vi "Controls and Indicators.vi"(4 "Motors Enable":bool[](array[boolean])=[FALSE, FALSE, FALSE], 5 "Virtual Spring":dbl=0.3, 6 "Tension Control":bool=TRUE, 7 "Velocity Damping":dbl=0.01, 8 "Start, End Point":bool[](array[boolean]), 9 "Target Stop":bool, 10 "Encoder Initialize":bool, 11 "Trajectory":i32(slide) scale=0.0..2.0) -> ()   [LabVIEW 2021]
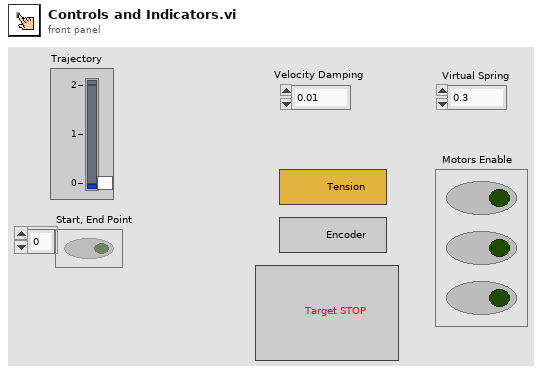
[diagram p1: front panel]
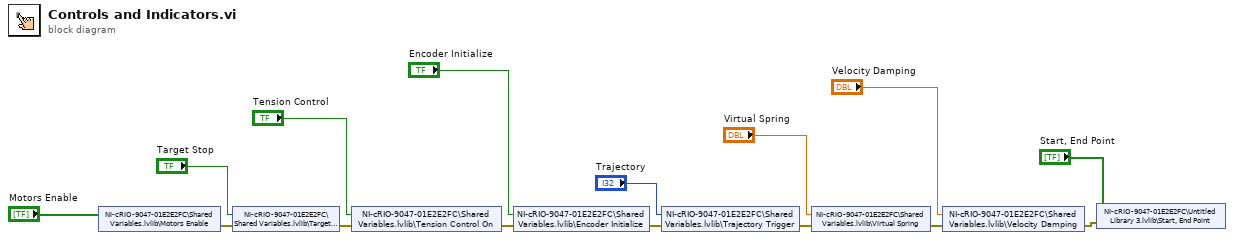
[diagram p0: block diagram]
diagram:
  n1 = shared-variable "NI-cRIO-9047-01E2E2FC\\Shared Variables.lvlib\\Motors Enable"("Motors Enable") -> (error out=w4:errorcluster)  [unwired: 1 in]
  n2 = shared-variable "NI-cRIO-9047-01E2E2FC\\Shared Variables.lvlib\\Target Stop"("Target Stop", error in=w4) -> (error out=w3:errorcluster)
  n3 = shared-variable "NI-cRIO-9047-01E2E2FC\\Shared Variables.lvlib\\Tension Control On"("Tension Control", error in=w3) -> (error out=w13:errorcluster)
  n4 = shared-variable "NI-cRIO-9047-01E2E2FC\\Shared Variables.lvlib\\Encoder Initialize"("Encoder Initialize", error in=w13) -> (error out=w14:errorcluster)
  n5 = shared-variable "NI-cRIO-9047-01E2E2FC\\Shared Variables.lvlib\\Trajectory Trigger"("Trajectory", error in=w14) -> (error out=w15:errorcluster)
  n6 = shared-variable "NI-cRIO-9047-01E2E2FC\\Shared Variables.lvlib\\Virtual Spring"("Virtual Spring", error in=w15) -> (error out=w12:errorcluster)
  n7 = shared-variable "NI-cRIO-9047-01E2E2FC\\Shared Variables.lvlib\\Velocity Damping"("Velocity Damping", error in=w12) -> (error out=w2:errorcluster)
  n8 = shared-variable "NI-cRIO-9047-01E2E2FC\\Untitled Library 3.lvlib\\Start, End Point"("Start, End Point", error in=w2) -> ()  [unwired: 1 out]
